vi "בדיקת זמן מיתוג הממסר Mod.vi"(7 "resultUserPrompt":bool, 8 "error":errorcluster, 9 "זמן מיתוג מקסימלי":dbl=0.03 format="%#_13g", 10 "שם הממסר":string="0410-24534 15A ממסר", 11 "Path for Log":path) -> (0 "error out":errorcluster, 1 "בטוח כן/לא":bool, 2 "בדיקת זמן מיתוג הממסר":dbl)   [LabVIEW 2015]
uses:
  <instrlib>/niDMM/nidmm.llb/niDMM Function.ctl
  <instrlib>/niDMM/nidmm.llb/niDMM Resolution in Digits.ctl
  <vilib>/DAQmx/write.llb/DAQmx Write (Digital Bool 1Line 1Point).vi
  <vilib>/DAQmx/create/channels.llb/DAQmx Create Channel (DO-Digital Output).vi
  <vilib>/DAQmx/miscellaneous.llb/DAQmx Fill In Error Info.vi
  <instrlib>/niDMM/nidmm.llb/niDMM Configure Measurement Digits.vi
panel:
  in  "התחל":bool
  # "Right-Click to\nexplain error"
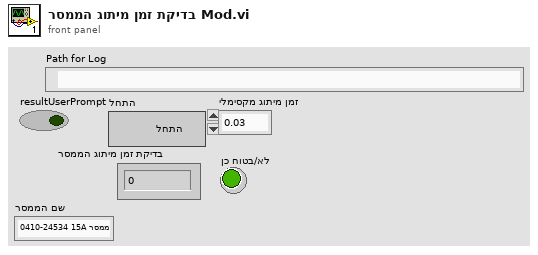
[diagram p1: front panel]
types:
  T1 = enum32{"Invalid", "Standard", "Closed", "Hidden", "Minimized", "Maximized"}
  T2 = typedef "niDMM Function.ctl" = enum16{"DC Volts", "AC Volts", "DC Current", "AC Current", "2-wire Resistance", "4-wire Resistance", "Diode", "Frequency", "Period", "AC Volts DC Coupled", "Capacitance", "Inductance", "Temperature"}
  T3 = typedef "niDMM Resolution in Digits.ctl" = dbl
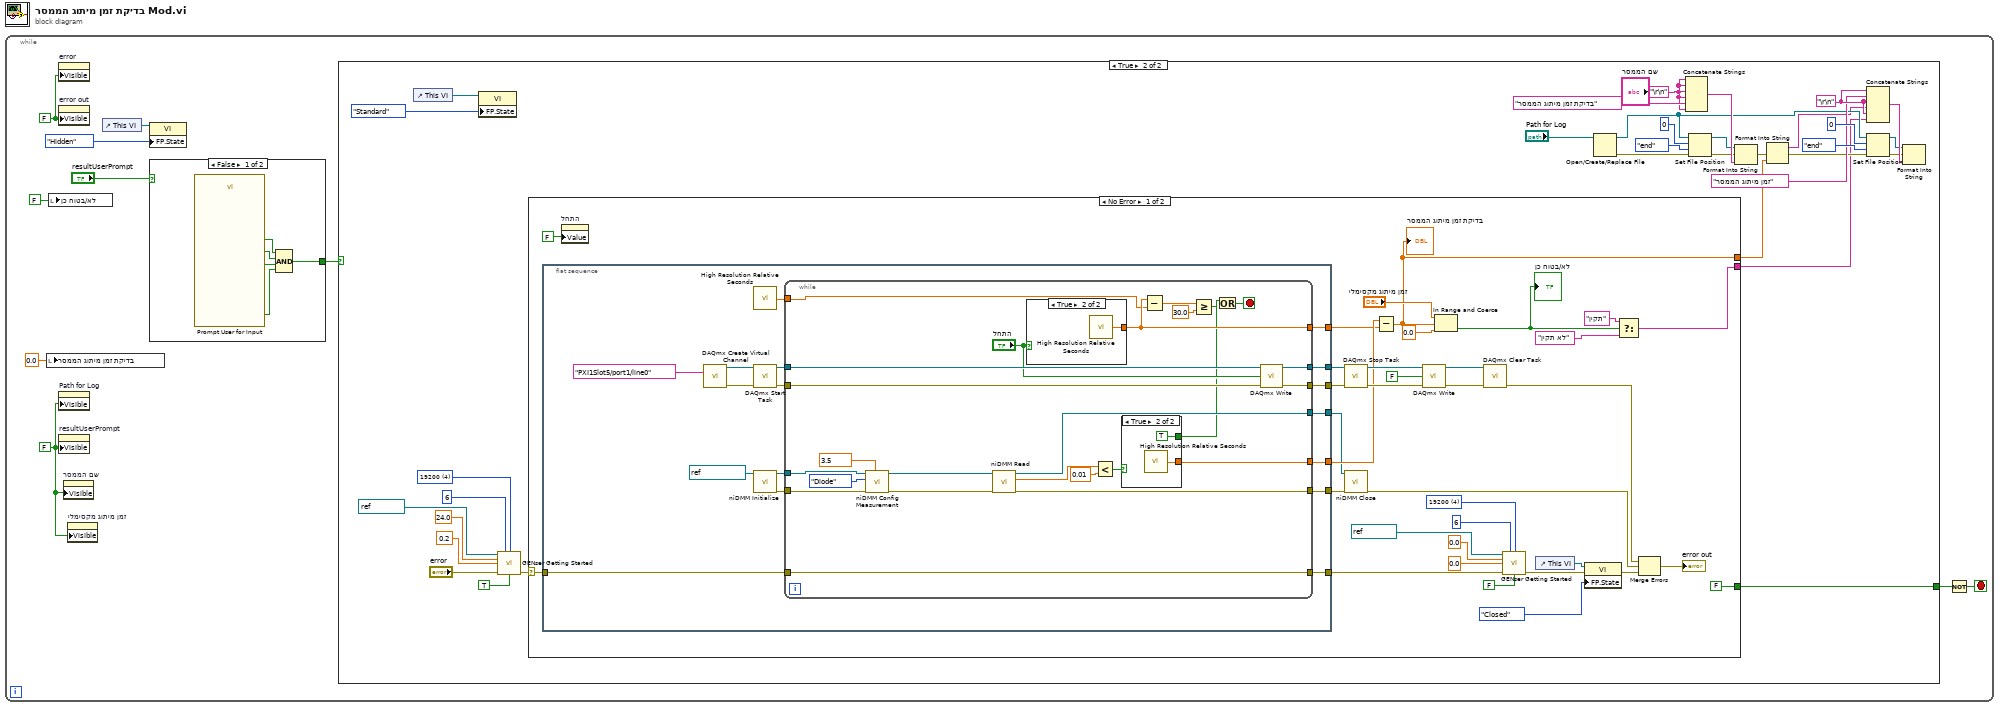
[diagram p0: block diagram]
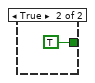
[diagram p2: hidden frame]
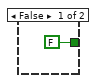
[diagram p3: hidden frame]
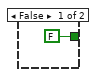
[diagram p4: hidden frame]
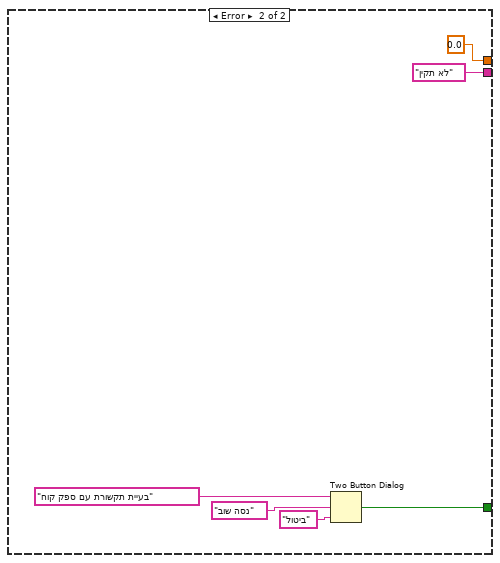
[diagram p6: hidden frame]
diagram:
  n1 = while {
    stop <- w8 stop-if-true
    w1 = FALSE ("Visible")
    w9 = FALSE ("Visible")
    n2 = local write "בדיקת זמן מיתוג הממסר"(0.0 ("בדיקת זמן מיתוג הממסר")) -> ()
    n3 = local write "בטוח כן/לא"(FALSE ("בטוח כן/לא")) -> ()
    n4 = property on="error" class="Clust (strict)"("Visible"=w9) -> ()  [unwired: 2 in, 2 out]
    n5 = property on="error out" class="Clust (strict)"("Visible"=w9) -> ()  [unwired: 2 in, 2 out]
    n6 = property on="Path for Log" class="Path"("Visible"=w1) -> ()  [unwired: 2 in, 2 out]
    n7 = property on="resultUserPrompt" class="Bool (strict)"("Visible"=w1) -> ()  [unwired: 2 in, 2 out]
    n8 = property on="שם הממסר" class="Str"("Visible"=w1) -> ()  [unwired: 2 in, 2 out]
    n9 = property on="זמן מיתוג מקסימלי" class="DigNum (strict)"("Visible"=w1) -> ()  [unwired: 2 in, 2 out]
    n10 = control-ref of="This VI"() -> (w7:refnum<vi>)
    n11 = property class="VI"(reference=w7, "FP.State"=T1."Hidden" ("Front Panel Window:State")) -> ()  [unwired: 1 in, 2 out]
    n12 = case shown="False" "resultUserPrompt" {
      tunnel: [w11 TRUE] -> w5
      frame False {
        n13 = call "Prompt User for Input"() -> ("הדקי הרב מודד"=w12:bool, "מגע שלילי"=w13:bool, "מגע חיובי"=w14:bool, "OK"=w15:bool)  [unwired: 15 in, 1 out]
        n14 = Compound Arithmetic op=AND(w15, w14, w13, w12) -> (w11:bool)
      }
      frame True {
      }
    }
    n15 = case shown="True" w5 {
      tunnel: [FALSE ("T button?") w44] -> w10
      frame False {
      }
      frame True {
        w27 = "\r\n"
        w34 = "\r\n"
        w47 = u16 4 items=["1200", "2400", "4800", "9600", "19200"] ("BAUD")
        n16 = control-ref of="This VI"() -> (w43:refnum<vi>)
        n17 = property class="VI"(reference=w43, "FP.State"=T1."Standard" ("Front Panel Window:State")) -> ()  [unwired: 1 in, 2 out]
        n18 = call "GENser Getting Started.vi"("VISA"=refnum<visa-resource-name> "COM6", "GEN Addr"=i16 6, "BAUD"=w47, "Voltage Limit"=24.0, "Current Limit"=0.2, "error"="error", "Output On (T)"=TRUE) -> ("error out"=w49:errorcluster)  [unwired: 5 in, 3 out]
        n19 = case shown="No Error" w49 {
          selector: w49 -> [w64 _]
          tunnel: [FALSE ("T button?") w135] -> w44
          tunnel: [w56 0.0] -> w19
          tunnel: [w52 "לא תקין"] -> w18
          frame No Error {
            w80 = u16 4 items=["1200", "2400", "4800", "9600", "19200"] ("BAUD")
            n20 = flat-sequence {
              tunnel: [w95] -> w70
              tunnel: [w94] -> w69
              tunnel: [w93] -> w68
              tunnel: [w92] -> w67
              tunnel: [w91] -> w66
              tunnel: [w90] -> w65
              tunnel: w64 -> [w89]
              tunnel: [w88] -> w63
              frame #0 {
                n21 = call-poly <vilib>:"DAQmx Create Virtual Channel.vi"("lines"=tag "PXI1Slot5/port1/line0") -> ("task out"=w99:refnum<k21>, "error out"=w100:errorcluster)  [unwired: 13 in]
                n22 = call <vilib>:"High Resolution Relative Seconds.vi"() -> ("relative seconds"=w87:dbl)
                n23 = call <vilib>:"DAQmx Start Task.vi"("task/channels in"=w99, "error in"=w100) -> ("task out"=w97:refnum<k21>, "error out"=w96:errorcluster)  [unwired: 12 in]
                n24 = call <instrlib>:"niDMM Initialize.vi"("Instrument Descriptor"=refnum<k15> "PXI1Slot9") -> ("error out"=w101:errorcluster, "instrument handle out"=w102:refnum<k15>)  [unwired: 9 in]
                n25 = while {
                  tunnel: [w111] -> w94
                  tunnel: [w126] -> w95
                  tunnel: [w115] -> w91
                  tunnel: [w125] -> w92
                  tunnel: [w124] -> w93
                  tunnel: [w114] -> w90
                  tunnel: w102 -> [w119]
                  tunnel: w101 -> [w118]
                  tunnel: w97 -> [w123]
                  tunnel: w96 -> [w122]
                  tunnel: [w113] -> w88
                  tunnel: w89 -> [w113]
                  tunnel: w87 -> [w110]
                  stop <- w107 stop-if-true
                  w128 = T3 3.5 items=["3 1/2"=3.5, "4 1/2"=4.5, "5 1/2"=5.5, "6 1/2"=6.5, "7 1/2"=7.5] ("Resolution in Digits")
                  n26 = call-poly <instrlib>:"niDMM Config Measurement.vi"("Resolution in Digits"=w128, "error in (no error)"=w118, "Function"=niDMM_Function."Diode", "instrument handle"=w119) -> ("error out"=w116:errorcluster, "instrument handle out"=w117:refnum<k15>)  [unwired: 6 in]
                  n27 = call <instrlib>:"niDMM Read.vi"("error in (no error)"=w116, "instrument handle"=w117) -> ("error out"=w114:errorcluster, "Measurement"=w121:dbl, "instrument handle out"=w115:refnum<k15>)  [unwired: 7 in]
                  n28 = case shown="True" "התחל" {
                    tunnel: [_ w132] -> w111
                    frame False {
                    }
                    frame True {
                      n29 = call <vilib>:"High Resolution Relative Seconds.vi"() -> ("relative seconds"=w132:dbl)
                    }
                  }
                  n30 = Less?(x=w121, y=0.01) -> (x < y?=w104:bool)
                  n31 = case shown="True" w104 {
                    tunnel: [_ w131] -> w126
                    tunnel: [FALSE TRUE] -> w106
                    frame False {
                    }
                    frame True {
                      n32 = call <vilib>:"High Resolution Relative Seconds.vi"() -> ("relative seconds"=w131:dbl)
                    }
                  }
                  n33 = Subtract(x=w111, y=w110) -> (x-y=w109:dbl)
                  n34 = Greater Or Equal?(x=w109, y=30.0) -> (x >= y?=w105:bool)
                  n35 = Or(x=w106, y=w105) -> (x .or. y?=w107:bool)
                  n36 = call-poly <vilib>:"DAQmx Write.vi"("task/channels in"=w123, "data"="התחל", "error in"=w122) -> ("task out"=w125:refnum<k21>, "error out"=w124:errorcluster)  [unwired: 10 in, 1 out]
                }
              }
            }
            n37 = property on="התחל" class="Bool (strict)"("Value"=FALSE ("data")) -> ()  [unwired: 2 in, 2 out]
            n38 = call <vilib>:"DAQmx Stop Task.vi"("task/channels in"=w67, "error in"=w68) -> ("task out"=w75:refnum<k21>, "error out"=w74:errorcluster)  [unwired: 12 in]
            n39 = call <instrlib>:"niDMM Close.vi"("error in (no error)"=w65, "instrument handle"=w66) -> ("error out"=w60:errorcluster)  [unwired: 9 in]
            n40 = Subtract(x=w70, y=w69) -> (x-y=w56:dbl)
            "בדיקת זמן מיתוג הממסר" <- w56
            n41 = call-poly <vilib>:"DAQmx Write.vi"("task/channels in"=w75, "data"=FALSE, "error in"=w74) -> ("task out"=w72:refnum<k21>, "error out"=w73:errorcluster)  [unwired: 10 in, 1 out]
            n42 = In Range and Coerce(upper limit="זמן מיתוג מקסימלי", x=w56, lower limit=0.0) -> (In Range?=w53:bool)  [unwired: 1 out]
            "בטוח כן/לא" <- w53
            n43 = call <vilib>:"DAQmx Clear Task.vi"("task in"=w72, "error in"=w73) -> ("error out"=w61:errorcluster)  [unwired: 13 in]
            n44 = call "GENser Getting Started.vi"("VISA"=refnum<visa-resource-name> "COM6", "GEN Addr"=i16 6, "BAUD"=w80, "Voltage Limit"=0.0, "Current Limit"=0.0, "error"=w63, "Output On (T)"=FALSE) -> ("error out"=w79:errorcluster)  [unwired: 5 in, 3 out]
            n45 = control-ref of="This VI"() -> (w78:refnum<vi>)
            n46 = property class="VI"(reference=w78, error in=w79, "FP.State"=T1."Closed" ("Front Panel Window:State")) -> (error out=w59:errorcluster)  [unwired: 1 out]
            n47 = Select(t="תקין", s=w53, f="לא תקין") -> (s? t:f=w52:string)
            n48 = Merge Errors(w61, w60, w59) -> (→"error out":errorcluster)
          }
          frame Error {
            n49 = Two Button Dialog(message="בעיית תקשורת עם ספק קוח", 1:"ביטול" ("F button name (\"Cancel\")"), 2:"נסה שוב" ("T button name (\"OK\")")) -> (T button?=w135:bool)
          }
        }
        n50 = Open/Create/Replace File(file path (use dialog)="Path for Log") -> (refnum out=w23:refnum<file>, error out=w24:errorcluster)  [unwired: 5 in, 1 out]
        n51 = Concatenate Strings(w34, w34, "שם הממסר", w34, "בדיקת זמן מיתוג הממסר", w34) -> (w38:string)
        n52 = Set File Position(offset (in bytes) (0)=i64 0, refnum=w23, from (0:start)=enum16{"start", "end", "current"}."end", error in=w24) -> (refnum out=w35:refnum<file>, error out=w33:errorcluster)
        n53 = Format Into String(initial string=w35, error in=w33, w38) -> (error out=w22:errorcluster)  [unwired: 1 in, 1 out]
        n54 = Format Into String(error in=w22, w19) -> (resulting string=w20:string, error out=w21:errorcluster)  [unwired: 2 in]
        n55 = Concatenate Strings(w27, "זמן מיתוג הממסר", w27, w20, w27, w18) -> (w32:string)
        n56 = Set File Position(offset (in bytes) (0)=i64 0, refnum=w23, from (0:start)=enum16{"start", "end", "current"}."end", error in=w21) -> (refnum out=w30:refnum<file>, error out=w31:errorcluster)
        n57 = Format Into String(initial string=w30, error in=w31, w32) -> ()  [unwired: 1 in, 2 out]
      }
    }
    n58 = Not(x=w10) -> (.not. x?=w8:bool)
  }
